vi "认识事件结构.vi"() -> ()   [LabVIEW 2018]
panel:
  in  "停止":bool
  out "字符串 2":string
  out "布尔":bool
  out "数值":dbl
  in  "旋钮":dbl(knob) scale=0.0..10.0
  in  "开机":bool
  in  "?":bool
  out "字符串":string="事件结构是在程序运行时可以通过前面板改变程序执行方式的结构\n类似中断响应"
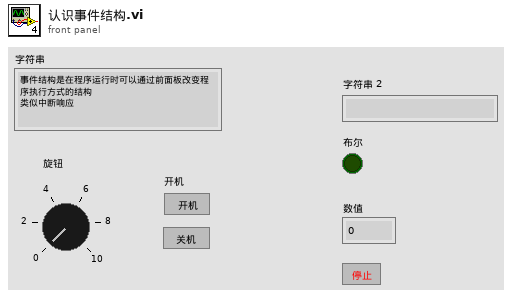
[diagram p1: front panel]
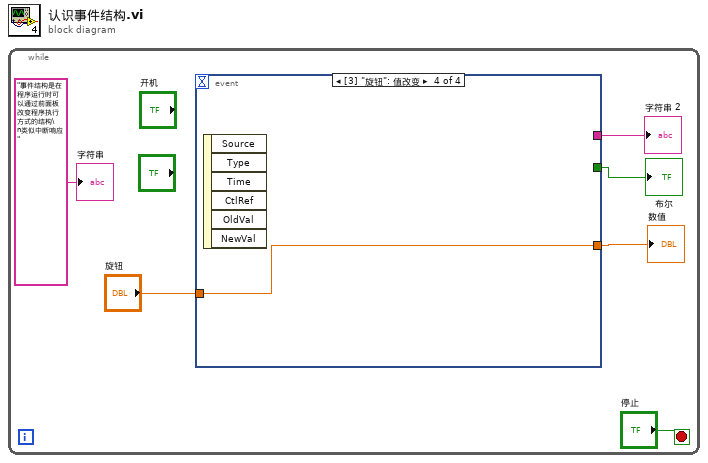
[diagram p0: block diagram]
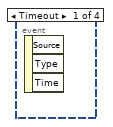
[diagram p2: hidden frame]
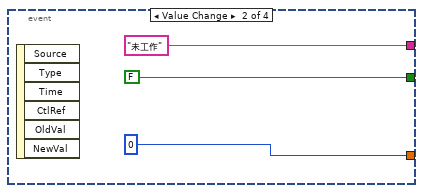
[diagram p3: hidden frame]
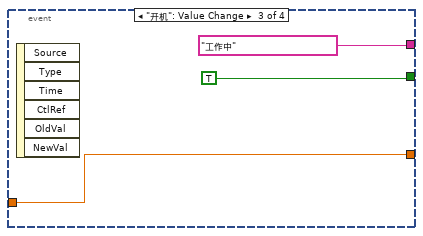
[diagram p4: hidden frame]
diagram:
  n1 = while {
    stop <- "停止" stop-if-true
    n2 = event shown="[3] \"旋钮\": 值改变" {
      selector: _ -> [_ _ _ _]
      dyn-events: _ -> [_ _ _ _]
      timeout: _ -> [_ _ _ _]
      tunnel: [_ "未工作" "工作中" _] -> w5
      tunnel: [_ FALSE TRUE _] -> w4
      tunnel: [_ 0 w10 w13] -> w1
      tunnel: "旋钮" -> [_ _ w10 w13]
      event Timeout {
        n3 = event-data() -> ()  [unwired: 1 in, 3 out]
      }
      event Value Change {
        n4 = event-data() -> ()  [unwired: 1 in, 6 out]
      }
      event "开机": Value Change {
        n5 = event-data() -> ()  [unwired: 1 in, 6 out]
      }
      event "旋钮": Value Change {
        n6 = event-data() -> ()  [unwired: 1 in, 6 out]
      }
    }
    "数值" <- w1
    "布尔" <- w4
    "字符串 2" <- w5
    "字符串" <- "事件结构是在程序运行时可以通过前面板改变程序执行方式的结构\n类似中断响应"
  }
